vi "Create.vi"(7 "Direction":T1, 8 "error in (no error)":errorcluster, 9 "Custom Config Data":u8[](array[numeric]), 10 "Name":string, 11 "CIFTag in":refnum<class "CIF_NIChn_FifoCAN.lvclass">) -> (0 "error out":errorcluster, 3 "CIFTag out":refnum<class "CIF_NIChn_FifoCAN.lvclass">)   [LabVIEW 2021, in "CIF_NIChn_FifoCAN.lvclass"]
uses:
  CIF_NIChn_FifoCAN.lvclass
  D:/dev/CIF-LVCore/src/Channels/CIFChannels/CIFChannels.lvclass
  D:/dev/CIF-LVCore/src/Channels/CIF_NIChn/NIChn/CIF_NIChnl.lvclass
  CIFChannels/Typedef/Direction.ctl
  CIFChannels/Typedef/Disconnect Behavior.ctl
  CIF_NIChn_FifoCAN.lvclass/CIF_NIChn_FifoCAN.ctl
  ChannelCommon/CIFFIFO/CIFfifo.lvclass/CIFfifo.ctl
  CIFChannels/CIFChannels.lvclass/CIFChannels.ctl
  CIFChannels/Typedef/Channel State.ctl
  NIChn/CIF_NIChn.lvclass/CIF_NIChn.ctl
  c6f1aac1-fdda-4143-8087-f9e7d57e6170.vi
  05c6e502-0377-480c-a15d-085597602460.vi
  CIFChannels/Accessors/Write Channel State.vi
  NIChn/Accessors/Write CIF Channel.vi
  CIFChannels/SubVIs/Get Type from Class.vi
  CIFChannels/Accessors/Write Type.vi
  CIFChannels/Accessors/Write Channel Class.vi
  CIFChannels/Accessors/Write Direction.vi
  CIFChannels/Accessors/Write Disconnect Behavior.vi
  CIFChannels/Accessors/Write Name.vi
  CIFChannels/Accessors/Write Custom Config Data.vi
  <vilib>/CIFChannels/SubVIs/Add Error.vi
  c6f1aac1-fdda-4143-8087-f9e7d57e6170.vi/c28b0ead-42ad-4072-80a2-aca7f2bd7ce3.vi
  <vilib>/CIFChannels/SubVIs/CIFServices Fill In Error Info Ex.vi
  <vilib>/CIFChannels/SubVIs/Get dll Path.vi
  c6f1aac1-fdda-4143-8087-f9e7d57e6170.vi/259f1102-a6f3-45ef-83a9-e8a266e5a7b9.vi
  05c6e502-0377-480c-a15d-085597602460.vi/c28b0ead-42ad-4072-80a2-aca7f2bd7ce3.vi
  ChannelCommon/Utilities/Unflatten FIFO Config.vi
  ChannelCommon/CIFFIFO/Accessors/Write Flags.vi
  <vilib>/CIFChannels/SubVIs/Append Error Location.vi
  ChannelCommon/Utilities/Expand FIFO Flags.vi
  <vilib>/Utility/LVClass/Get LV Class Name.vi
  CIFChannels/CIFChannels.lvclass
  ChannelCommon/CIFFIFO/CIFfifo.lvclass
  D:/dev/CIF-LVCore/src/Channels/CIF_NIChn/NIChn/CIF_NIChn.lvclass
  D:/dev/CIF-LVCore/src/Channels/CIF_NIChn/FIFO_CAN/CIF_NIChn_FifoCAN.lvclass
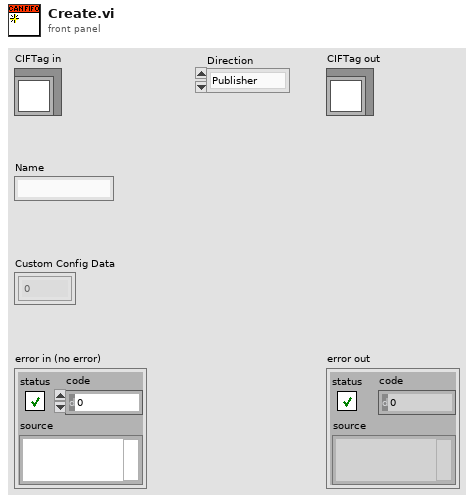
[diagram p1: front panel]
types:
  T1 = typedef "CIFChannels.lvclass/Direction.ctl" = enum16{"Publisher", "Subscriber"}
  T2 = typedef "CIFChannels.lvclass/Disconnect Behavior.ctl" = enum16{"Default value", "Last value", "Error with default"}
  T3 = typedef "CIFChannels.lvclass/Channel State.ctl" = enum16{"Creating", "Disconnected", "Connecting", "Connected", "Destroyed"}
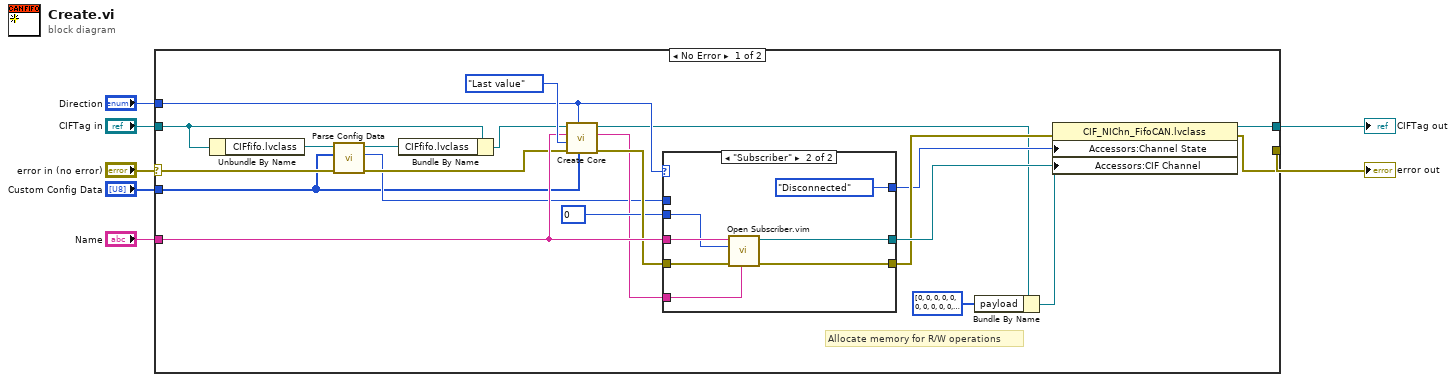
[diagram p0: block diagram]
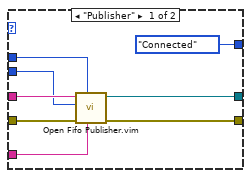
[diagram p2: hidden frame]
diagram:
  n1 = case shown="No Error" "error in (no error)" {
    selector: "error in (no error)" -> [w11 w46]
    tunnel: [w28 w46] -> w6
    tunnel: [w22 w45] -> w4
    tunnel: "CIFTag in" -> [w14 w45]
    tunnel: "Name" -> [w27 _]
    tunnel: "Direction" -> [w21 _]
    tunnel: "Custom Config Data" -> [w8 _]
    frame No Error {
      # "Allocate memory for R/W operations"
      n2 = Unbundle By Name(w14) -> ("CIFfifo.lvclass"=w13:refnum<class "CIFfifo.lvclass">)
      n3 = call "Parse Config Data.vi"("error in (no error)"=w11, "Custom Config Data"=w8, "CIFfifo in"=w13) -> ("error out"=w10:errorcluster, "Depth"=w9:u64, "CIFfifo out"=w12:refnum<class "CIFfifo.lvclass">)  [unwired: 6 in]
      n4 = Bundle By Name(cluster=w14, "CIFfifo.lvclass"=w12) -> (w17:refnum<class "CIF_NIChn_FifoCAN.lvclass">)
      n5 = call "Create Core.vi"("Custom Config Data"=w8, "Direction"=w21, "error in (no error)"=w10, "Disconnect Behavior"=Disconnect_Behavior."Last value", "Name"=w27, "CIFChannels in"=w17) -> ("error out"=w26:errorcluster, "Channel Type"=w15:string, "CIFChannels out"=w19:refnum<class "CIF_NIChn_FifoCAN.lvclass">)  [unwired: 3 in]
      n6 = case shown="\"Subscriber\"" w21 {
        tunnel: w27 -> [w37 w43]
        tunnel: w26 -> [w36 w42]
        tunnel: [w32 w38] -> w25
        tunnel: [w33 w39] -> w23
        tunnel: w15 -> [w35 w41]
        tunnel: [Channel_State."Connected" ("Channel State") Channel_State."Disconnected" ("Channel State")] -> w20
        tunnel: u8 0 -> [w31 w40]
        tunnel: w9 -> [w30 _]
        frame "Publisher" {
          n7 = call "Open Fifo Publisher.vim"("Channel Type Description"=w35, "depth"=w30, "error in"=w36, "Input Type"=w31, "Channel Name"=w37) -> ("error out"=w33:errorcluster, "CIF Channel"=w32:refnum<k21>)  [unwired: 5 in]
        }
        frame "Subscriber" {
          n8 = call "Open Subscriber.vim"("Channel Type Description"=w41, "error in"=w42, "Input Type"=w40, "Channel Name"=w43) -> ("error out"=w39:errorcluster, "CIF Channel"=w38:refnum<k21>)  [unwired: 6 in]
        }
      }
      n9 = Bundle By Name(cluster=w19, "payload"=u8[] [0, 0, 0, 0, 0, 0, 0, 0, 0, 0, 0, 0, 0, 0, 0, 0, 0, 0, 0, 0, 0, 0, 0, 0, 0, 0, 0, 0, 0, 0, 0, 0, 0, 0, 0, 0, 0, 0, 0, 0, 0, 0, 0, 0, 0, 0, 0, 0, 0, 0, 0, 0, 0, 0, 0, 0, 0, 0, 0, 0, 0, 0, 0, 0, 0, 0, 0, 0, 0, 0, 0, 0, 0, 0, 0, 0, 0, 0, 0, 0, 0, 0, 0, 0, 0, 0, 0, 0, 0, 0, 0, 0, 0, 0, 0, 0, 0, 0, 0, 0, 0, 0, 0, 0, 0, 0, 0, 0, 0, 0, 0, 0, 0, 0, 0, 0, 0, 0, 0, 0, 0, 0, 0, 0, 0, 0, 0, 0, 0, 0, 0, 0, 0, 0, 0, 0, 0, 0, 0, 0, 0, 0, 0, 0, 0, 0, 0, 0, 0, 0, 0]) -> (w24:refnum<class "CIF_NIChn_FifoCAN.lvclass">)
      n10 = property class="CIF_NIChn_FifoCAN.lvclass"(reference=w24, error in=w23, "Accessors:Channel State"=w20, "Accessors:CIF Channel"=w25) -> (reference out=w22:refnum<class "CIF_NIChn_FifoCAN.lvclass">, error out=w28:errorcluster)
    }
    frame Error {
    }
  }
  "error out" <- w6
  "CIFTag out" <- w4
